vi "Read SwitchACIR Channel.vi"(8 "error in (no error)":errorcluster, 11 "SwitchACIR configuration":refnum<class "SwitchACIR Channel configuration.lvclass">) -> (0 "error out":errorcluster, 2 "SwitchACIR Channel":T1, 3 "SwitchACIR configuration out":refnum<class "SwitchACIR Channel configuration.lvclass">)   [LabVIEW 2025, in "SwitchACIR Channel configuration.lvclass"]
uses:
  SwitchACIR Channel configuration.lvclass
  SwitchACIR Channel Setting.ctl
  SwitchACIR Channel configuration.lvclass/SwitchACIR Channel configuration.ctl
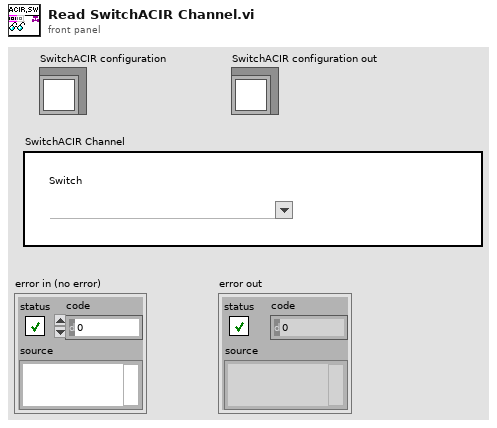
[diagram p1: front panel]
types:
  T1 = typedef "SwitchACIR Channel configuration.lvclass/SwitchACIR Channel Setting.ctl" = cluster{"Switch":string}
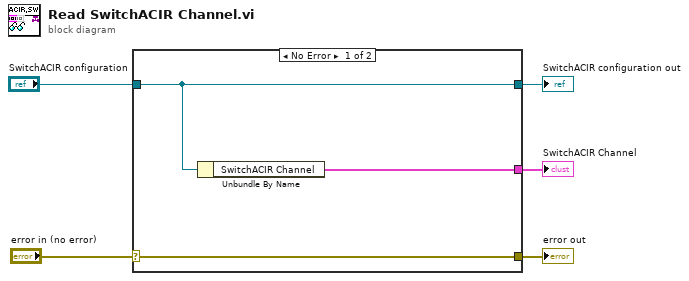
[diagram p0: block diagram]
diagram:
  n1 = case shown="No Error" "error in (no error)" {
    selector: "error in (no error)" -> [w8 w9]
    tunnel: [w8 w9] -> w4
    tunnel: [w7 w10] -> w2
    tunnel: "SwitchACIR configuration" -> [w7 w10]
    tunnel: [w6 _] -> w1
    frame No Error {
      n2 = Unbundle By Name(w7) -> ("SwitchACIR Channel"=w6:T1)
    }
    frame Error {
    }
  }
  "error out" <- w4
  "SwitchACIR configuration out" <- w2
  "SwitchACIR Channel" <- w1
